vi "OE2011&OE2021_Configure Auto Range.vi"(7 "OE2011&OE2021_\nAuto Range":T1={"Auto Gain"=FALSE, "Signal In Channel"=1} {"Signal In Channel" items=["Signal In1"=1]}, 8 "Error in (no error)":errorcluster caption="error out（no error）", 9 "Remote Mode":u16(ring) items=["USB", "RS232", "GPIB", "Ethernet"], 10 "Connection ID in":refnum<k5>, 11 "VISA resource name":refnum<visa-resource-name>) -> (0 "Error out":errorcluster caption="error out", 1 "Output String":string, 2 "Connection ID out":refnum<k5>, 3 "VISA resource  out":refnum<visa-resource-name>)   [LabVIEW 2011]
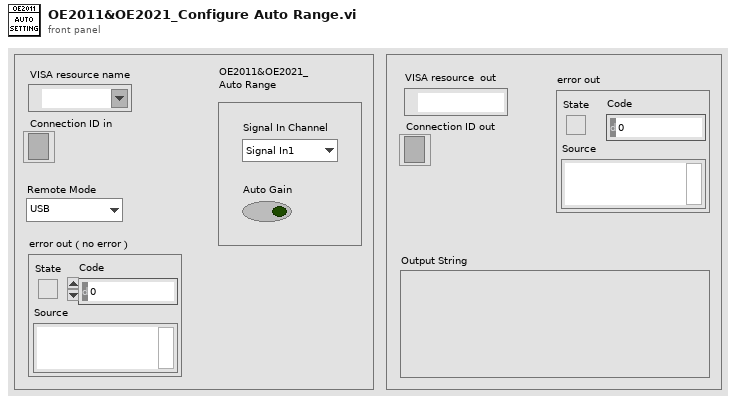
[diagram p1: front panel]
types:
  T1 = cluster{"Auto Gain":bool, "Signal In Channel":u16}
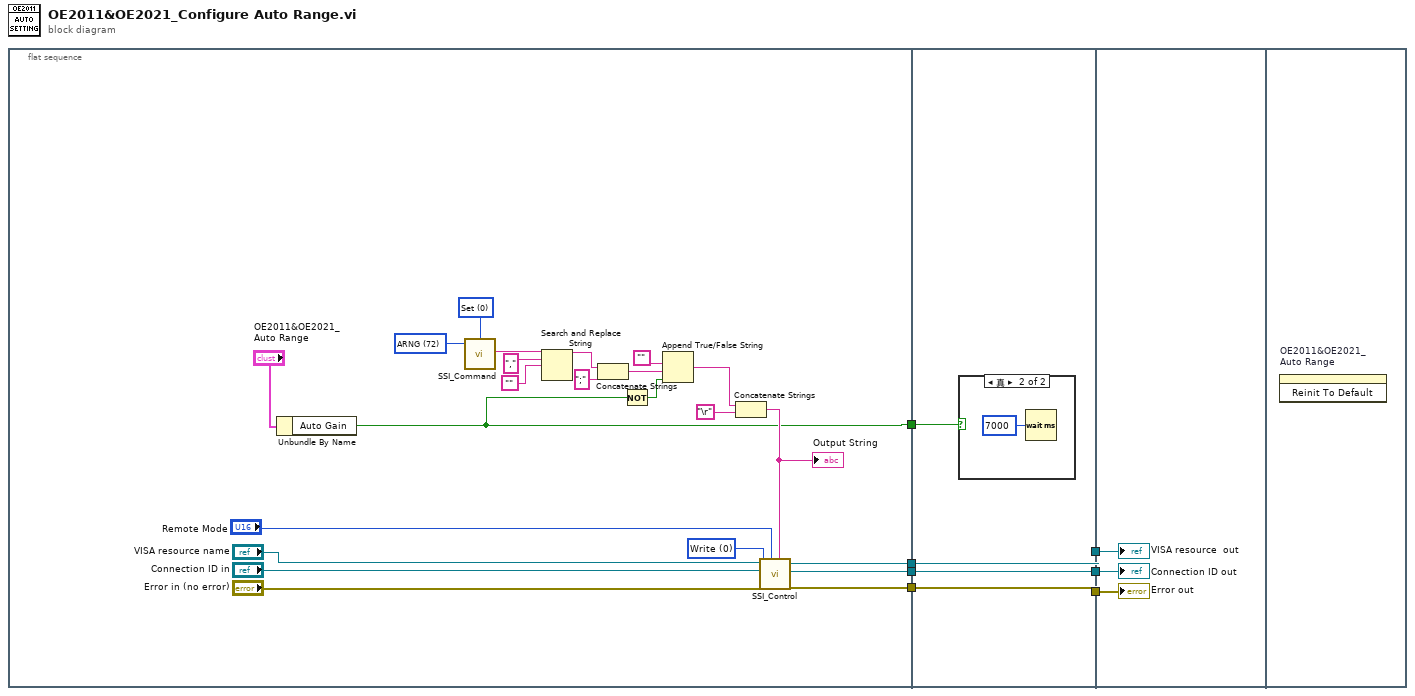
[diagram p0: block diagram]
diagram:
  n1 = flat-sequence {
    tunnel: [w26] -> w7
    tunnel: [w25] -> w6
    tunnel: [w24] -> w5
    tunnel: [w8] -> w1
    tunnel: w7 -> [w34]
    tunnel: w6 -> [w33]
    tunnel: w5 -> [w32]
    tunnel: [w34] -> w4
    tunnel: [w33] -> w3
    tunnel: [w32] -> w2
    tunnel: w1 -> [w31]
    tunnel: w4 -> [w37]
    tunnel: w3 -> [w38]
    tunnel: w2 -> [w36]
    frame #0 {
      w13 = u16 72 items=["ISRC", "IGND", "ICPL", "ILIN", "PHAS", "FMOD", "RSLP", "FREQ", "SWPT", "SLLM", "SULM", "SSLL", "SSLG", "STLM", "SWRM", "IRNG", "SENS", "RMOD", "OFLT", "OFSL", "SYNC", "DMOD", "HARM", "DARB", "SWVT", "SLVL", "SVLL", "SVUL", "SVSL", "SVSG", "SVTM", "SVRM", "RALL", "SNAP", "OUTP", "OAUX", "COUT", "CAUX", "COFP", "CEXP", "FPOP", "OEXP", "*IDN", "*RST", "OVLD", "INOV", "GNOV", "*PLL", "SSET", "RSET", "AGAN", "APHS", "ARSV", "ASCL", "EQCD", "EQCS", "SPED", "SRAT", "SLEN", "SSLE", "STRG", "SPRM", "STRD", "PAUS", "REST", "SPTS", "TRCA", "TEMP", "RSTU", "INHZ", "DEQU", "SADD", "ARNG", "CSPE", "ISRCD", "IGNDD", "ICPLD", "ILIND", "PHASD", "FMODD", "RSLPD", "FREQD", "SWPTD", "SLLMD", "SULMD", "SSLLD", "SSLGD", "STLMD", "SWRMD", "SENSD", "RMODD", "OFLTD", "OFSLD", "SYNCD", "HARMD", "EQCDD", "EQCSD", "SNAPD", "OUTPD", "SWVTD", "SLVLD", "SVLLD", "SVULD", "SVSLD", "SVSGD", "SVTMD", "SVRMD", "SVDCD", "ARSVD", "AGAND", "APHSD", "ASCLD", "FPOPD", "CAUXD", "OEXPD", "SPEDD", "SRATD", "SLEND", "SSLED", "STRGD", "SPRMD", "STRDD", "PAUSD", "RESTD", "SPTSD", "TRCAD", "*IDND", "*RSTD", "INOVD", "GNOVD", "*PLLD", "SSETD", "RSETD", "RALLD", "NIPA", "NSMA", "NGWA", "NMAC", "NMOD", "TRIG", "TRCB", "INHZD", "ISAMD", "IRAGD", "RRAGD", "SOFFD", "DMODD", "COUTD", "COFPD", "CEXPD", "ARNGD", "OAUXD", "TRIM", "SUITD", "SNHZD", "AOFSD", "RSRC", "FEXT", "FINT", "DSRC", "DARF", "DEAF", "DREF", "SSRC", "STTL", "SIGO", "SLVL", "SOFF", "SPHS", "TPHS", "SMOD", "MARF", "AMSR", "AMDP", "FMSR", "FMDV", "PMSR", "PMDV", "CHDC", "AUXV", "AFLT", "AOFP"] ("Command Type")
      w14 = u16 0 items=["Set", "Query"] ("Opera")
      w27 = u16 0 items=["Write", "Read"] ("Control")
      n2 = Unbundle By Name("OE2011&OE2021_\nAuto Range") -> ("Auto Gain"=w8:bool)
      n3 = call "SSI_Command.vi"("Opera"=w14, "Command Type"=w13) -> ("Output string"=w17:string)  [unwired: 2 in]
      n4 = Search and Replace String(input string=w17, search string="," ("搜索字符串"), replace string="") -> (result string=w19:string)  [unwired: 5 in, 3 out]
      n5 = Concatenate Strings(w19, ";") -> (w18:string)
      n6 = Not(x=w8) -> (.not. x?=w9:bool)
      n7 = Append True/False String(1:w9, 2:w18, 3:"") -> (0:w15:string)  [unwired: 1 in]
      n8 = Concatenate Strings(w15, "\r") -> (w10:string)
      "Output String" <- w10
      n9 = call "SSI_Control.vi"("Write Buffer"=w10, "Remote Mode"="Remote Mode", "Error in (no error)"="Error in (no error)", "Control"=w27, "Connection ID in"="Connection ID in", "VISA resource name"="VISA resource name") -> ("Error out"=w24:errorcluster, "Connection ID out"=w26:refnum<k5>, "VISA resource  out"=w25:refnum<visa-resource-name>)  [unwired: 2 in, 1 out]
    }
    frame #1 {
      n10 = case shown="真" w31 {
        frame False {
        }
        frame True {
          n11 = Wait (ms)(milliseconds to wait=u32 7000 ("等待时间（毫秒）")) -> ()  [unwired: 1 out]
        }
      }
    }
    frame #2 {
      "Error out" <- w36
      "Connection ID out" <- w37
      "VISA resource  out" <- w38
    }
    frame #3 {
      n12 = invoke on="OE2011&OE2021_\nAuto Range" class="Clust (严格)" method="Reinit To Default"() -> ()  [unwired: 3 in, 3 out]
    }
  }
